vi "Initialize Time Register.vi"(7 "Sample rate (Hz)":u32, 8 "error in (no error)":errorcluster, 10 "Name":string, 11 "FPGA Ref":refnum<k20>) -> (0 "error out":errorcluster, 3 "FPGA Ref out":refnum<k20>)   [LabVIEW 2019, in "Fuel Injector Analysis Addon Engine.lvlib"]
uses:
  Fuel Injector Analysis Addon Engine.lvlib
  <vilib>/NI/LVFPGA Adv Session Resources/OpenByNameSubVI.vi
  <vilib>/rvi/interface/common/dynamic/niFpgaEscapeDelimiterAndNull.vi
  <vilib>/Utility/error.llb/Error Cluster From Error Code.vi
  <vilib>/rvi/errors/niLvFpgaAdjustHostInterfaceError.vi
  <vilib>/FPGAPlugInAG/Dynamic/niLvFpga_Close_Dynamic.vi
  <vilib>/NI/LVFPGA Adv Session Resources/OpenByName.xnode
  <vilib>/rvi/interface/nirviReadWriteControl/nirviReadWriteControl.xnode
  <vilib>/rvi/interface/nirviCloseFPGA/nirviCloseFPGA.xnode
  <vilib>/rvi/interface/Simulation/niFpgaSimulationCallBeginRW.vi
  NiFpgaLv.dll
  <vilib>/NI/LVFPGA Adv Session Resources/LVFPGAAdvSessionResources.lvlib
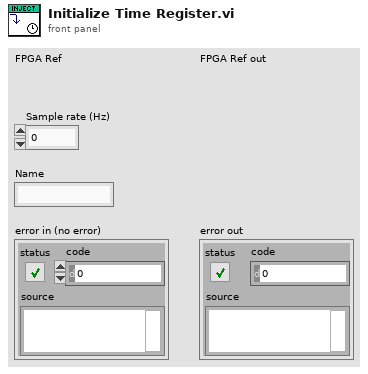
[diagram p1: front panel]
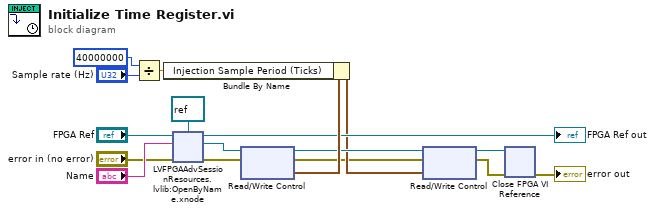
[diagram p0: block diagram]
diagram:
  n1 = Divide(x=u32 40000000 ("y"), y="Sample rate (Hz)") -> (x/y=w17:dbl)
  n2 = xnode "LVFPGAAdvSessionResources.lvlib:OpenByName.xnode"("FPGA VI Reference in"="FPGA Ref", "Resource name in"="Name", "Single resource reference type in"=refnum<k20> refnum ("Injector.Timing"), "Error in"="error in (no error)") -> ("Single resource reference out"=w5:refnum<k20>, "Error out"=w6:errorcluster, "FPGA VI Reference out"=→"FPGA Ref out":refnum<k20>)
  n3 = xnode "Read/Write Control"("FPGA VI Reference In"=w5, "error in"=w6) -> ("FPGA VI Reference Out"=w4:refnum<k20>, "error out"=w1:errorcluster, "Value"=w14:cluster{"Injection Sample Period (Ticks)":u32})
  n4 = Bundle By Name(cluster=w14, "Injection Sample Period (Ticks)"=w17) -> (w2:cluster{"Injection Sample Period (Ticks)":u32})
  n5 = xnode "Read/Write Control"("FPGA VI Reference In"=w4, "error in"=w1, "Value"=w2) -> ("FPGA VI Reference Out"=w11:refnum<k20>, "error out"=w12:errorcluster)
  n6 = xnode "Close FPGA VI Reference"("FPGA VI Reference In"=w11, "error in"=w12) -> ("error out"=→"error out":errorcluster)
